vi "Read Channel Groups Decimation Values.vi"(8 "error in":errorcluster, 11 "channel groups in":T1[](array[typedef]) {"Decimation Ref" format="%.0x"; "Block Refs"."Data Reference" format="%.0x"}) -> (0 "error out":errorcluster, 2 "channel groups decimations":i32[](array[numeric]), 3 "channel groups out":T1[](array[typedef]) {"Decimation Ref" format="%.0x"; "Block Refs"."Data Reference" format="%.0x"})   [LabVIEW 2027, in "Embedded Data Logger Engine.lvlib"]
uses:
  Embedded Data Logger Engine.lvlib
  Group Sampling Specification.ctl
  <vilib>/NI VeriStand/Custom Device API/Block Data Reference.ctl
  <vilib>/NI VeriStand/Custom Device API/Data Reference.ctl
  <vilib>/NI VeriStand/Custom Device API/Custom Device API.lvlib
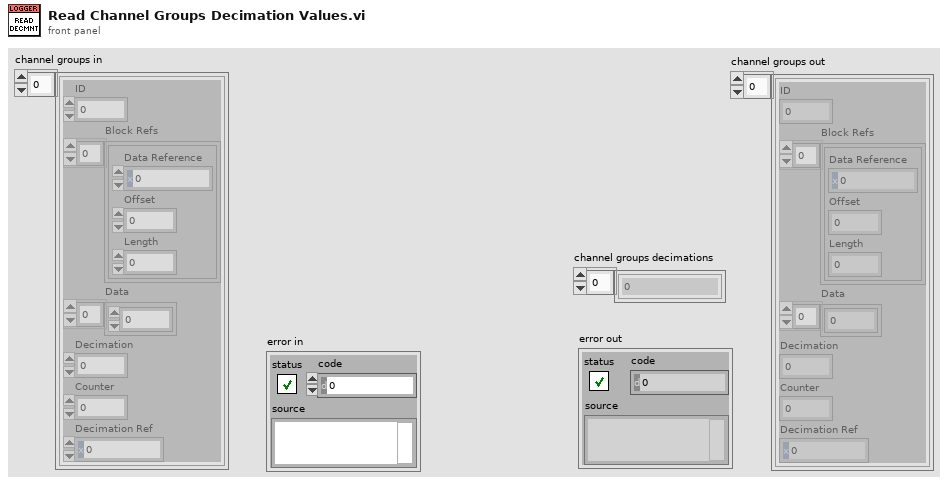
[diagram p1: front panel]
types:
  T1 = typedef "Embedded Data Logger Engine.lvlib/Group Sampling Specification.ctl" = cluster{"ID":dbl, "Block Refs":T2[], "Data":dbl[], "Decimation":i32, "Counter":i32, "Decimation Ref":T3}
  T2 = typedef "Custom Device API.lvlib/Block Data Reference.ctl" = cluster{"Data Reference":T3, "Offset":u64, "Length":u64}
  T3 = typedef "Custom Device API.lvlib/Data Reference.ctl" = i32
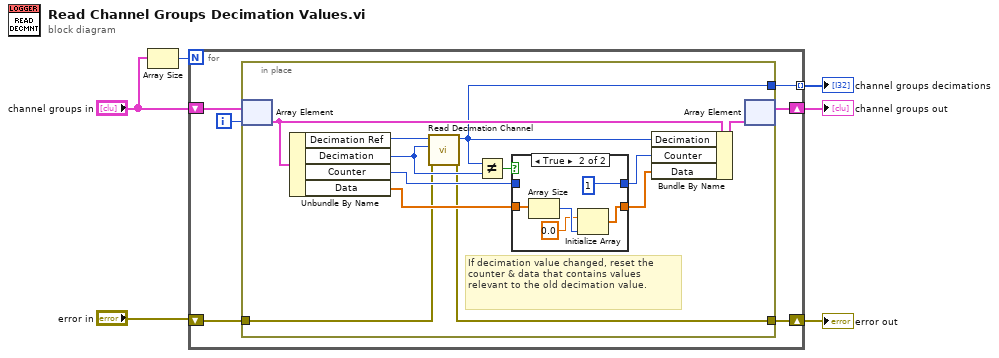
[diagram p0: block diagram]
diagram:
  n1 = Array Size(array="channel groups in") -> (size(s)=w4:i32)
  n2 = for {
    N: w4 -> [_]
    shift-right: [w11] -> w6
    shift-left: "channel groups in" -> [w12]
    tunnel: [w9] -> w5 mode=indexing
    shift-right: [w7] -> w1
    shift-left: "error in" -> [w8]
    i -> [w10]
    n3 = in-place {
      in-place-border: [w21] -> w9
      in-place-border: w8 -> [w15]
      in-place-border: [w14] -> w7
      # "If decimation value changed, reset the counter & data that contains values relevant to the old decimation value."
      n4 = in-place-array #1(w12, w10) -> (w23:T1)
      n5 = Unbundle By Name(w23) -> ("Decimation Ref"=w22:T3, "Decimation"=w20:i32, "Counter"=w18:i32, "Data"=w19:dbl[])
      n6 = call "Read Decimation Channel.vi"("error in"=w15, "default decimation"=w20, "decimation reference in"=w22) -> ("error out"=w14:errorcluster, "decimation"=w21:i32)  [unwired: 7 in]
      n7 = Not Equal?(x=w21, y=w20) -> (x != y?=w13:bool)
      n8 = case shown="True" w13 {
        tunnel: [w26 1 ("t")] -> w17
        tunnel: w18 -> [w26 _]
        tunnel: w19 -> [w25 w30]
        tunnel: [w25 w27] -> w16
        frame False {
        }
        frame True {
          n9 = Array Size(array=w30) -> (size(s)=w29:i32)
          n10 = Initialize Array(0.0 ("element"), w29) -> (w27:dbl[])
        }
      }
      n11 = Bundle By Name(cluster=w23, "Decimation"=w21, "Counter"=w17, "Data"=w16) -> (w24:T1)
      n12 = in-place-array #1(w24) -> (w11:T1[])  [unwired: 1 out]
    }
  }
  "error out" <- w1
  "channel groups out" <- w6
  "channel groups decimations" <- w5
